vi "VCS Read Position Marker Counter.vi"(8 "error in (no error)":errorcluster, 11 "axis in":cluster{"keyHandle":u32, "nodeId":u16}={"keyHandle"=0, "nodeId"=1}) -> (0 "error out":errorcluster, 1 "count":u16, 3 "axis out":cluster{"keyHandle":u32, "nodeId":u16}={"keyHandle"=0, "nodeId"=1})   [LabVIEW 2017, in "maxonEPOS.lvlib"]
doc: "<B>VCS_ReadPositionMarkerCounter</B> returns the number of the detected edges."
uses:
  Examples/maxonEPOS.lvlib
  SSI_Tool/InstrumentsInterfaces/Motordriver/maxon EPOS/Resources/EposCmd.dll
  SSI_Tool/InstrumentsInterfaces/Motordriver/maxon EPOS/Resources/EposCmd64.dll
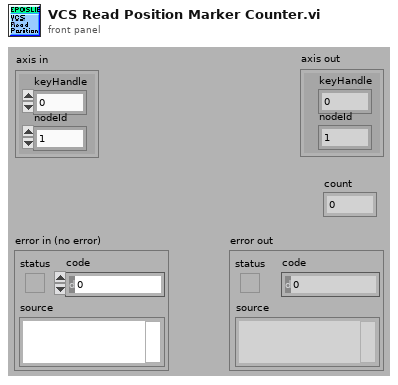
[diagram p1: front panel]
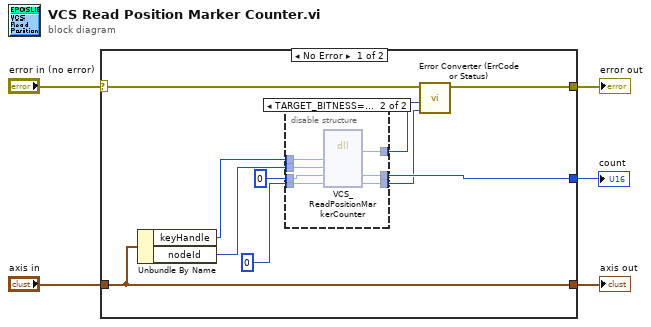
[diagram p0: block diagram]
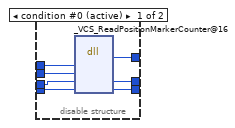
[diagram p2: hidden frame]
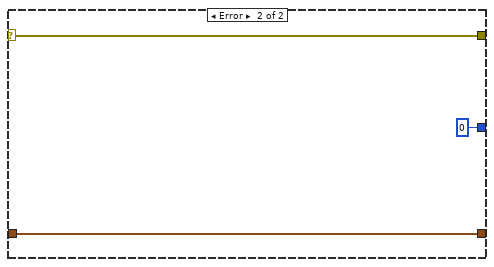
[diagram p3: hidden frame]
diagram:
  n1 = case shown="No Error" "error in (no error)" {
    selector: "error in (no error)" -> [w13 w31]
    tunnel: "axis in" -> [w15 w32]
    tunnel: [w15 w32] -> w4
    tunnel: [w14 w31] -> w3
    tunnel: [w12 u16 0 ("pCount")] -> w1
    frame No Error {
      n2 = Unbundle By Name(w15) -> ("keyHandle"=w6:u32, "nodeId"=w7:u16)
      n3 = disable-structure shown="TARGET_BITNESS==64" {
        disable-tunnel: [w22 w29] -> w12
        disable-tunnel: [w21 w28] -> w11
        disable-tunnel: [w20 w27] -> w10
        disable-tunnel: u32 0 ("pErrorCode") -> [w19 w26]
        disable-tunnel: u16 0 ("pCount") -> [w18 w25]
        disable-tunnel: w7 -> [w17 w24]
        disable-tunnel: w6 -> [w16 w23]
        frame condition #0 (active) {
          n4 = dll-call lib="C:/workspace/project/scancon/sw/SSI_Tool/InstrumentsInterfaces/Motordriver/maxon EPOS/Resources/EposCmd.*" fn="_VCS_ReadPositionMarkerCounter@16"("KeyHandle"=w16, "NodeId"=w17, "pCount"=w18, "pErrorCode"=w19) -> (w21:i32, "pCount"=w22:u16, "pErrorCode"=w20:u32)  [unwired: 5 in, 2 out]
        }
        frame condition #1 {
          n5 = dll-call lib="C:/setup/Resources/EposCmd64.*" fn="VCS_ReadPositionMarkerCounter" ("EposCmd.dll:_VCS_ReadPositionMarkerCounter@16")("KeyHandle"=w23, "NodeId"=w24, "pCount"=w25, "pErrorCode"=w26) -> ("Rückgabetyp"=w28:i32, "pCount"=w29:u16, "pErrorCode"=w27:u32)  [unwired: 5 in, 2 out]
        }
      }
      n6 = call "Error Converter (ErrCode or Status).vi"("error code"=w10, "return type"=w11, "error in (no error)"=w13) -> ("error out"=w14:errorcluster)  [unwired: 7 in]
    }
    frame Error {
    }
  }
  "count" <- w1
  "error out" <- w3
  "axis out" <- w4
